vi "Solve1.vi"(8 "Error In":errorcluster, 11 "object in":refnum<class "2022_1.lvclass">) -> (0 "Error Out":errorcluster, 2 "Result":u64, 3 "object out":refnum<class "2022_1.lvclass">)   [LabVIEW 2020, in "2022_1.lvclass"]
uses:
  2022_1.lvclass
  2022_1.lvclass/2022_1.ctl
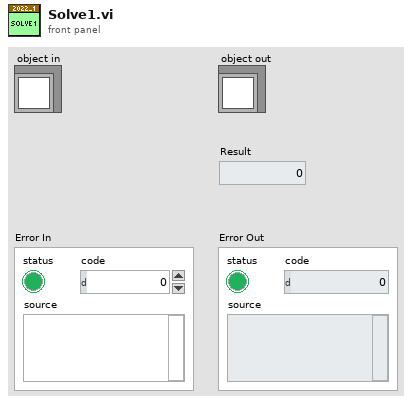
[diagram p1: front panel]
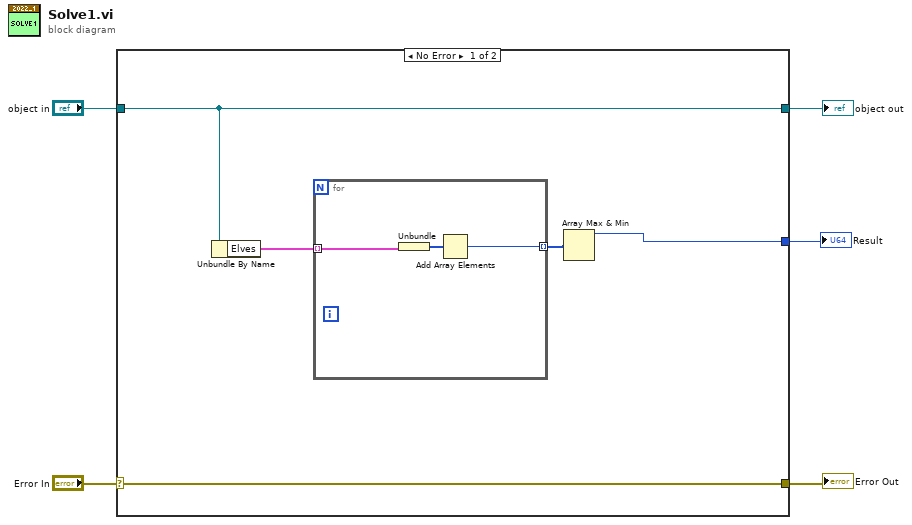
[diagram p0: block diagram]
diagram:
  n1 = case shown="No Error" "Error In" {
    selector: "Error In" -> [w10 w15]
    tunnel: [w10 w15] -> w4
    tunnel: [w9 w14] -> w2
    tunnel: "object in" -> [w9 w14]
    tunnel: [w6 _] -> w1
    frame No Error {
      n2 = Unbundle By Name(w9) -> ("Elves"=w8:cluster{"Calories":u64[]}[])
      n3 = for {
        tunnel: w8 -> [w13] mode=indexing
        tunnel: [w11] -> w7 mode=indexing
        n4 = Unbundle(w13) -> ("Calories"=w12:u64[])
        n5 = Add Array Elements(numeric array=w12) -> (sum=w11:u64)
      }
      n6 = Array Max & Min(array=w7) -> (max value=w6:u64)  [unwired: 3 out]
    }
    frame Error {
    }
  }
  "Error Out" <- w4
  "object out" <- w2
  "Result" <- w1
